vi "Error Table.vi"(11 "Error in":errorcluster) -> (4 "Error Table":string[][](table), 15 "Error out":errorcluster)   [LabVIEW 2020]
doc: "This VI is used as a error log VI which is used to get the errors which are generated due to the current and voltage values not falling in the required limit"
uses:
  Typedefs/Stop cases.ctl
panel:
  in  "Stop":bool
  # "Error Log"
  # "Press to terminate\nexecution"
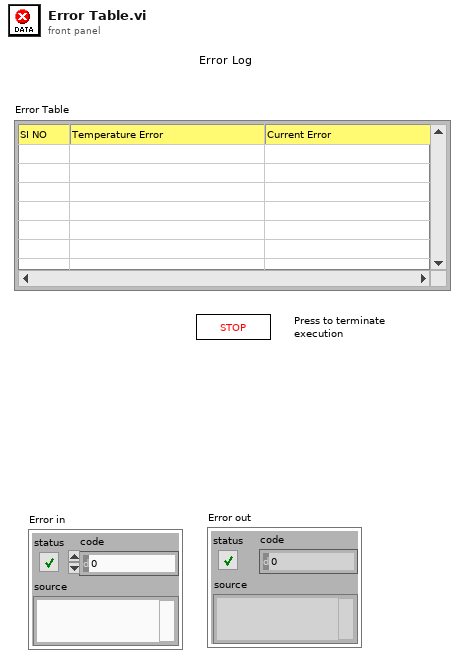
[diagram p1: front panel]
types:
  T1 = typedef "Stop cases.ctl" = enum16{"Initialize", "Write", "Stop"}
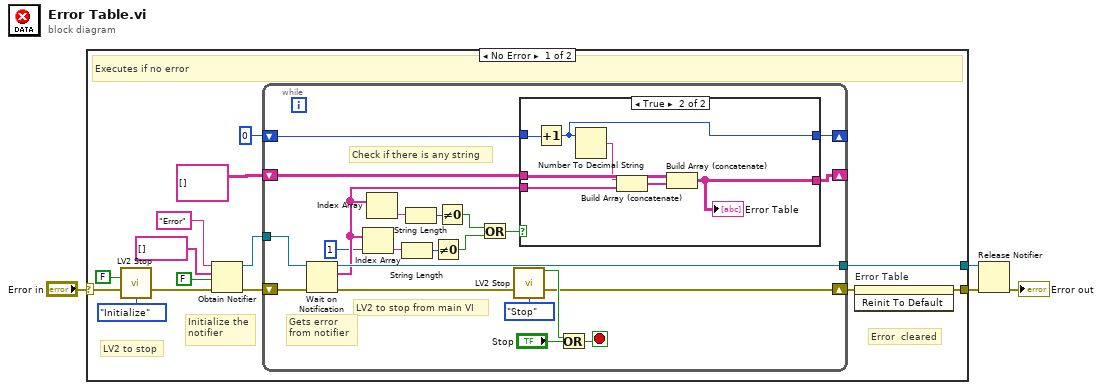
[diagram p0: block diagram]
diagram:
  n1 = case shown="No Error" "Error in" {
    selector: "Error in" -> [w10 w50]
    tunnel: [w7 w50] -> w3
    tunnel: [w5 _] -> w1
    frame No Error {
      # "Error  cleared"
      # "Initialize the \nnotifier"
      # "LV2 to stop"
      # "Executes if no error"
      n2 = call "LV2 Stop.vi"("Stop"=FALSE, "Error in"=w10, "Operation"=Stop_cases."Initialize") -> ("Error out"=w9:errorcluster)  [unwired: 11 in, 1 out]
      n3 = Obtain Notifier(name (unnamed)="Error", notification data type=string[] [], create if not found? (T)=FALSE, error in (no error)=w9) -> (notifier out=w14:refnum<notifier>, error out=w16:errorcluster)  [unwired: 1 out]
      n4 = while {
        tunnel: w14 -> [w39]
        shift-right: [w29] -> _
        shift-left: string[][] [] -> [w38]
        shift-right: [w26] -> w8
        shift-left: w16 -> [w40]
        shift-right: [w28] -> _
        shift-left: 0 -> [w30]
        tunnel: [w27] -> w5
        stop <- w34 stop-if-true
        # "Check if there is any string"
        # "LV2 to stop from main VI"
        # "Gets error\nfrom notifier"
        n5 = Wait on Notification(notifier=w39, error in (no error)=w40) -> (notifier out=w27:refnum<notifier>, notification=w23:string[], error out=w37:errorcluster)  [unwired: 2 in, 1 out]
        n6 = Index Array(array=w23, index=1) -> (element=w25:string)
        n7 = Index Array(array=w23) -> (element=w32:string)  [unwired: 1 in]
        n8 = String Length(string=w25) -> (length=w24:i32)
        n9 = String Length(string=w32) -> (length=w31:i32)
        n10 = Not Equal To 0?(x=w24) -> (x != 0?=w20:bool)
        n11 = Not Equal To 0?(x=w31) -> (x != 0?=w21:bool)
        n12 = Or(x=w21, y=w20) -> (x .or. y?=w22:bool)
        n13 = call "LV2 Stop.vi"("Error in"=w37, "Operation"=Stop_cases."Stop") -> ("Output"=w33:bool, "Error out"=w26:errorcluster)  [unwired: 12 in]
        n14 = case shown="True" w22 {
          tunnel: w38 -> [w41 w49]
          tunnel: w23 -> [_ w48]
          tunnel: w30 -> [w42 w46]
          tunnel: [w41 w44] -> w29
          tunnel: [w42 w43] -> w28
          frame False {
          }
          frame True {
            n15 = Increment(x=w46) -> (x+1=w43:i32)
            n16 = Number To Decimal String(number=w43) -> (decimal integer string=w45:string)  [unwired: 1 in]
            n17 = Build Array (concatenate)(w45, w48) -> (w47:string[])
            n18 = Build Array (concatenate)(w49, w47) -> (w44:string[][])
            "Error Table" <- w44
          }
        }
        n19 = Or(x=w33, y="Stop") -> (x .or. y?=w34:bool)
      }
      n20 = invoke on="Error Table" class="Tbl (strict)" method="Reinit To Default"(error in=w8) -> (error out=w7:errorcluster)  [unwired: 2 in, 2 out]
    }
    frame Error {
      # "Terminates execution if there is error"
    }
  }
  n21 = Release Notifier(notifier=w1, error in (no error)=w3) -> (error out=→"Error out":errorcluster)  [unwired: 1 in, 2 out]
